vi "Dynamic call-message window.vi"(8 "error in (no error)":errorcluster, 11 "Message":string) -> (0 "error out":errorcluster)   [LabVIEW 2013]
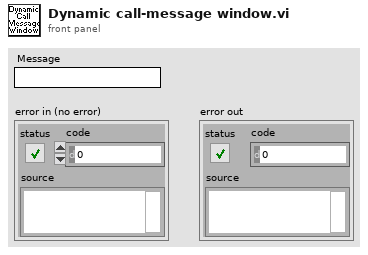
[diagram p1: front panel]
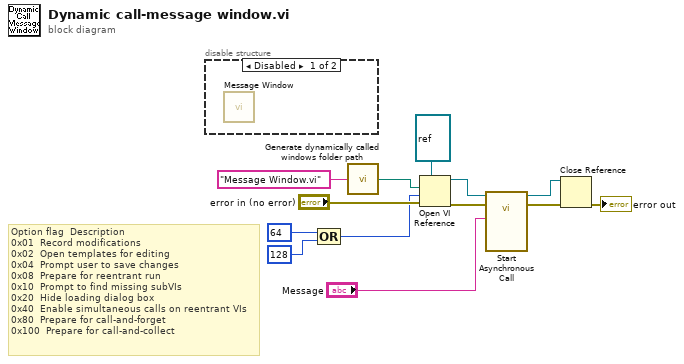
[diagram p0: block diagram]
diagram:
  # "Option flag \tDescription\n0x01 \tRecord modifications\n0x02 \tOpen templates for editing\n0x04 \tPrompt user to save changes\n0x08 \tPrepare for reentrant run\n0x10 \tPrompt to find missing subVIs\n0x20 \tHide loading dialog box\n0x40 \tEnable simultaneous calls on reentrant VIs\n0x80 \tPrepare for call-and-forget\n0x100 \tPrepare for call-and-collect"
  n1 = disable-structure shown="Disabled" {
    frame Disabled {
      n2 = call "Message Window.vi"() -> ()  [unwired: 11 in, 1 out]
    }
    frame Enabled {
    }
  }
  n3 = Compound Arithmetic op=OR(64, 128) -> (w6:i32)
  n4 = call "Generate dynamically called windows folder path.vi"("name of dynamically called VI"="Message Window.vi" ("Error Source")) -> ("Dynamically called VI path"=w10:path)
  n5 = Open VI Reference(type specifier VI Refnum (for type only)=refnum<vi> refnum, vi path=w10, options=w6, error in (no error)="error in (no error)") -> (vi reference=w7:refnum<vi>, error out=w8:errorcluster)  [unwired: 2 in]
  n6 = call-by-ref "Start Asynchronous Call"(reference=w7, error in=w8, "Message string"="Message") -> (reference out=w1:refnum<vi>, error out=w2:errorcluster)  [unwired: 10 in, 1 out]
  n7 = Close Reference(reference=w1, error in (no error)=w2) -> (error out=→"error out":errorcluster)
